vi "LS370 Change Excitation text out.vi"(4 "extra wait":i32, 6 "Current":u16, 7 "Channel":i32=1 min=1 max=16 step=1, 9 "Mode":enum32{"Voltage", "Current"}(ring), 10 "Resistance Range":T1, 11 "VISA Refnum in":refnum<visa-resource-name>) -> (3 "Command text":string[][](array[string]))   [LabVIEW 2025]
doc: "Author: Scott Hannahs <sth@magnet.fsu.edu>\n\nThis software is licensed for use under the “MIT License\"\nCopyright (c) 2025 Scott Hannahs, sth@sth@magnet.sthnet.net\n\nPermission is hereby granted, free of charge, to any person obtaining a copy of this software and associated documentation files (the \"Software\"), to deal in the Software without restriction, including without limitation the rights to use, copy, modify, merge, publish, distribute, sublicense, and/or sell copies of the Software, and to permit persons to whom the Software is furnished to do so, subject to the following conditions: The above copyright notice and this permission notice shall be included in all copies or substantial portions of the Software.\n\nTHE SOFTWARE IS PROVIDED \"AS IS\", WITHOUT WARRANTY OF ANY KIND, EXPRESS OR IMPLIED, INCLUDING BUT NOT LIMITED TO THE WARRANTIES OF MERCHANTABILITY, FITNESS FOR A PARTICULAR PURPOSE AND NONINFRINGEMENT. IN NO EVENT SHALL THE AUTHORS OR COPYRIGHT HOLDERS BE LIABLE FOR ANY CLAIM, DAMAGES OR OTHER LIABILITY, WHETHER IN AN ACTION OF CONTRACT, TORT OR OTHERWISE, ARISING FROM, OUT OF OR IN CONNECTION WITH THE SOFTWARE OR THE USE OR OTHER DEALINGS IN THE SOFTWARE."
uses:
  LS370 Resistance Range.ctl
  LS370 Excitation Voltage.ctl
  LS370 Excitation Current.ctl
panel:
  out "action description":string
  # "Address"
  # "Command"
  # "Descrtption"
  # "Extra Wait"
  # "R range"
  # "Mode"
  # "Device"
  # "Wait until"
  # "Wait before"
  # "Excitation"
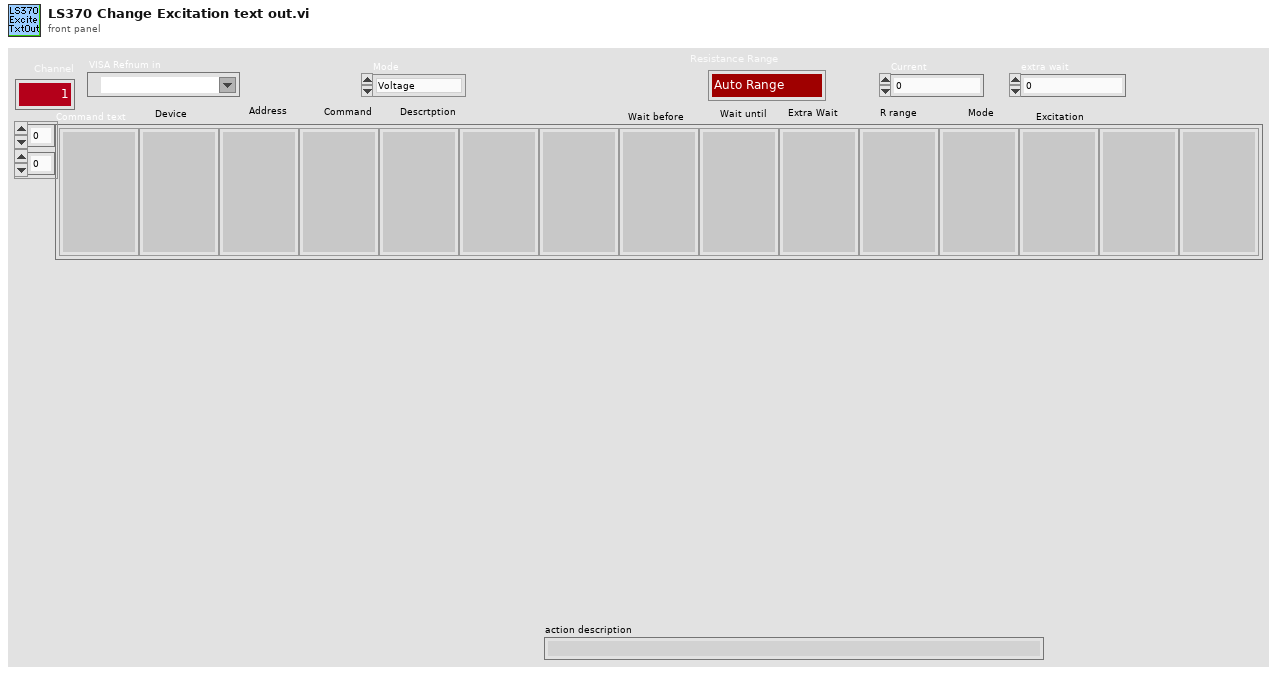
[diagram p1: front panel]
types:
  T1 = typedef "LS370 Resistance Range.ctl" = enum16{"Auto Range", "2.00 mΩ", "6.32 mΩ", "20.0 mΩ", "63.2 mΩ", "200 mΩ", "632 mΩ", "2.00 Ω", "6.32 Ω", "20.0 Ω", "63.2 Ω", "200 Ω", "632 Ω", "2.00 kΩ", "6.32 kΩ", "20.0 kΩ", "63.2 kΩ", "200 kΩ", "632 kΩ", "2.00 MΩ", "6.32 MΩ", "20.0 MΩ", "63.2 MΩ"}
  T2 = typedef "LS370 Excitation Voltage.ctl" = enum16{"2.00 µV", "6.32 µV", "20.0 µV", "63.2 µV", "200 µV", "632 µV", "2.00 mV", "6.32 mV", "20.0 mV", "63.2 mV", "200 mV", "632 mV"}
  T3 = typedef "LS370 Excitation Current.ctl" = enum16{"1.00 pA", "3.16 pA", "10.0 pA", "31.6 pA", "100 pA", "316 pA", "1.00 nA", "3.16 nA", "10.0 nA", "31.6 nA", "100 nA", "316 nA", "1.00 µA", "3.16 µA", "10.0 µA", "31.6 µA", "100 µA", "316 µA", "1.00 mA", "3.16mA", "10.0 mA", "31.6 mA"}
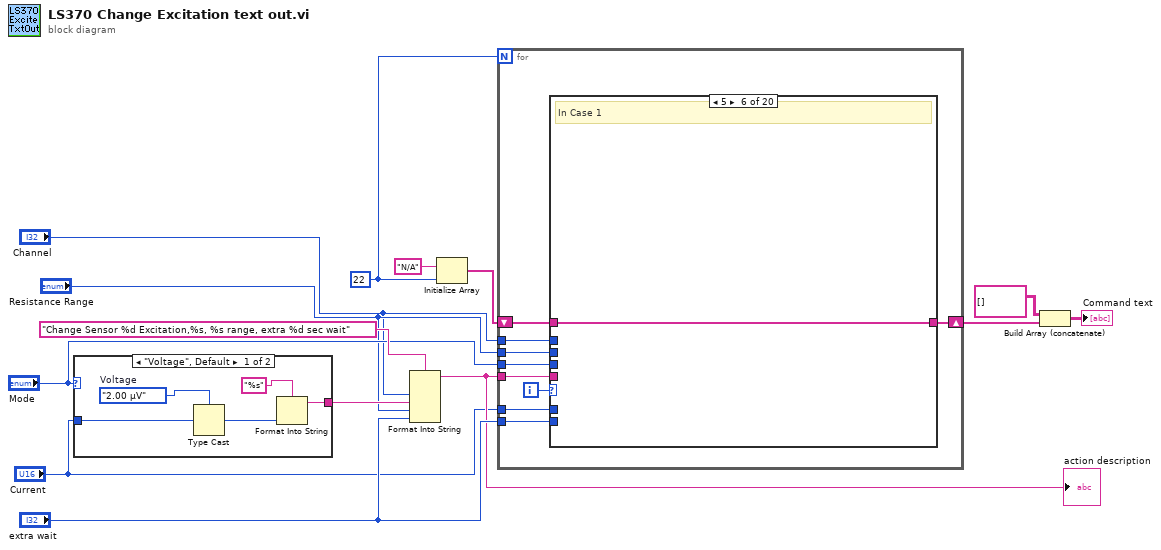
[diagram p0: block diagram]
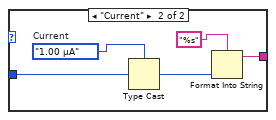
[diagram p2: hidden frame]
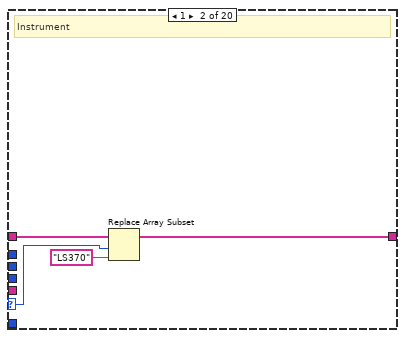
[diagram p4: hidden frame]
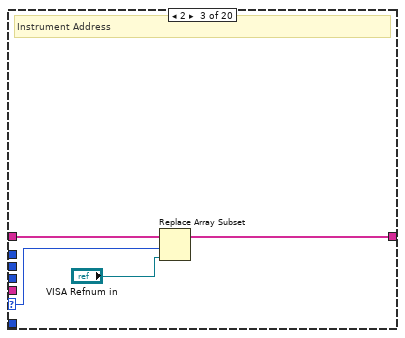
[diagram p5: hidden frame]
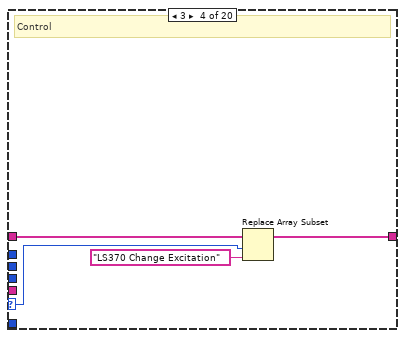
[diagram p6: hidden frame]
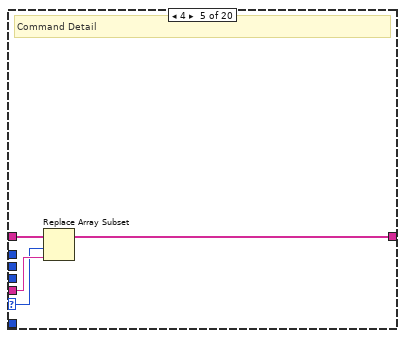
[diagram p7: hidden frame]
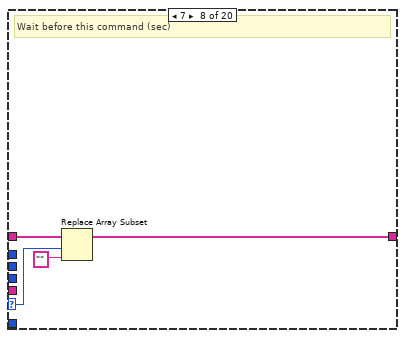
[diagram p9: hidden frame]
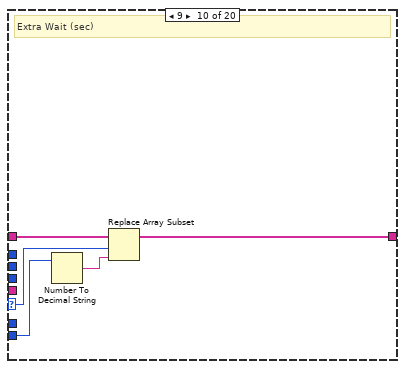
[diagram p11: hidden frame]
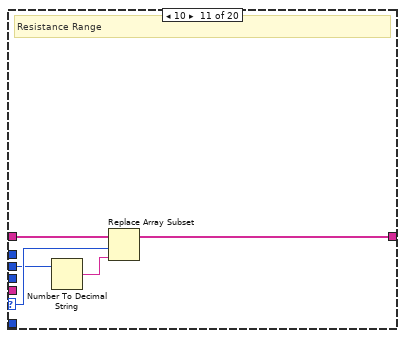
[diagram p12: hidden frame]
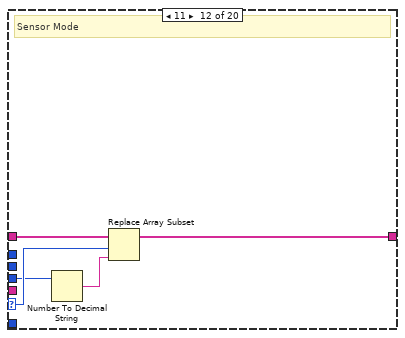
[diagram p13: hidden frame]
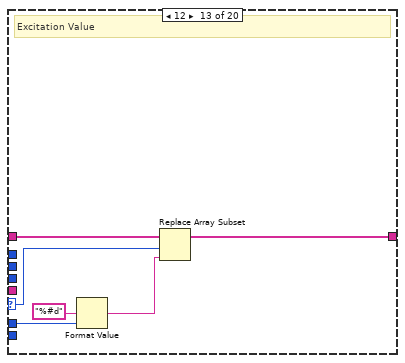
[diagram p14: hidden frame]
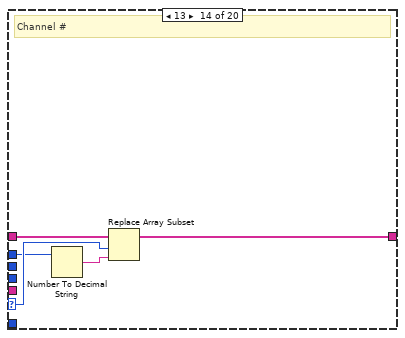
[diagram p15: hidden frame]
diagram:
  w13 = 22
  n1 = case shown="\"Voltage\", Default" "Mode" {
    tunnel: "Current" -> [w19 w24]
    tunnel: [w17 w22] -> w8
    frame "Voltage", Default {
      w15 = LS370_Excitation_Voltage."2.00 µV"  # Voltage
      n2 = Type Cast(type=w15, x=w19) -> (*(type *) &x=w18:T2)
      n3 = Format Into String(format string="%s", w18) -> (resulting string=w17:string)  [unwired: 2 in, 1 out]
    }
    frame "Current" {
      w20 = LS370_Excitation_Current."1.00 µA"  # Current
      n4 = Type Cast(type=w20, x=w24) -> (*(type *) &x=w23:T3)
      n5 = Format Into String(format string="%s", w23) -> (resulting string=w22:string)  [unwired: 2 in, 1 out]
    }
  }
  n6 = Format Into String(format string="Change Sensor %d Excitation,%s, %s range, extra %d sec wait", "Channel", w8, "Resistance Range", "extra wait") -> (resulting string=w6:string)  [unwired: 2 in, 1 out]
  "action description" <- w6
  n7 = Initialize Array("N/A", w13) -> (w12:string[])
  n8 = for {
    N: w13 -> [_]
    shift-right: [w30] -> w10
    shift-left: w12 -> [w32]
    tunnel: w6 -> [w31]
    tunnel: "extra wait" -> [w29]
    tunnel: "Mode" -> [w28]
    tunnel: "Current" -> [w27]
    tunnel: "Resistance Range" -> [w26]
    tunnel: "Channel" -> [w25]
    i -> [w33]
    n9 = case shown="5" w33 {
      selector: w33 -> [_ w35 w40 w43 w47 _ _ w53 _ w58 w65 w69 w74 w80 _ _ _ _ _ _]
      tunnel: w32 -> [w34 w37 w42 w45 w50 w51 w52 w56 w57 w62 w66 w71 w78 w82 w84 w85 w86 w87 w88 w89]
      tunnel: w31 -> [_ _ _ _ w49 _ _ _ _ _ _ _ _ _ _ _ _ _ _ _]
      tunnel: [w34 w36 w41 w44 w48 w51 w52 w55 w57 w61 w67 w72 w77 w81 w84 w85 w86 w87 w88 w89] -> w30
      tunnel: w29 -> [_ _ _ _ _ _ _ _ _ w59 _ _ _ _ _ _ _ _ _ _]
      tunnel: w28 -> [_ _ _ _ _ _ _ _ _ _ _ w68 _ _ _ _ _ _ _ _]
      tunnel: w27 -> [_ _ _ _ _ _ _ _ _ _ _ _ w73 _ _ _ _ _ _ _]
      tunnel: w26 -> [_ _ _ _ _ _ _ _ _ _ w64 _ _ _ _ _ _ _ _ _]
      tunnel: w25 -> [_ _ _ _ _ _ _ _ _ _ _ _ _ w79 _ _ _ _ _ _]
      frame 0, Default {
        # "Line #"
      }
      frame 1 {
        # "Instrument"
        n10 = Replace Array Subset(array=w37, new element="LS370", index=w35) -> (w36:string[])
      }
      frame 2 {
        # "Instrument Address"
        n11 = Replace Array Subset(array=w42, new element="VISA Refnum in", index=w40) -> (w41:string[])
      }
      frame 3 {
        # "Control"
        n12 = Replace Array Subset(array=w45, new element="LS370 Change Excitation", index=w43) -> (w44:string[])
      }
      frame 4 {
        # "Command Detail"
        n13 = Replace Array Subset(array=w50, new element=w49, index=w47) -> (w48:string[])
      }
      frame 5 {
        # "In Case 1"
      }
      frame 6 {
        # "In Case 2"
      }
      frame 7 {
        # "Wait before this command (sec)"
        n14 = Replace Array Subset(array=w56, new element="" ("new element/subarray"), index=w53) -> (w55:string[])
      }
      frame 8 {
        # "Wait Until the Action is finished? 1=yes 0=no"
      }
      frame 9 {
        # "Extra Wait (sec)"
        n15 = Number To Decimal String(number=w59) -> (decimal integer string=w60:string)  [unwired: 1 in]
        n16 = Replace Array Subset(array=w62, new element=w60, index=w58) -> (w61:string[])
      }
      frame 10 {
        # "Resistance Range"
        n17 = Number To Decimal String(number=w64) -> (decimal integer string=w63:string)  [unwired: 1 in]
        n18 = Replace Array Subset(array=w66, new element=w63, index=w65) -> (w67:string[])
      }
      frame 11 {
        # "Sensor Mode"
        n19 = Number To Decimal String(number=w68) -> (decimal integer string=w70:string)  [unwired: 1 in]
        n20 = Replace Array Subset(array=w71, new element=w70, index=w69) -> (w72:string[])
      }
      frame 12 {
        # "Excitation Value"
        n21 = Format Value(format string="%#d", value (0)=w73) -> (output string=w76:string)  [unwired: 1 in]
        n22 = Replace Array Subset(array=w78, new element=w76, index=w74) -> (w77:string[])
      }
      frame 13 {
        # "Channel #"
        n23 = Number To Decimal String(number=w79) -> (decimal integer string=w83:string)  [unwired: 1 in]
        n24 = Replace Array Subset(array=w82, new element=w83, index=w80) -> (w81:string[])
      }
      frame 14 {
      }
      frame 15 {
      }
      frame 16 {
      }
      frame 17 {
      }
      frame 18 {
      }
      frame 19 {
      }
    }
  }
  n25 = Build Array (concatenate)(string[][] [], w10) -> (→"Command text":string[][])
